vi "Init Sim Starter Kit.vi"(8 "error in (no error)":errorcluster, 10 "robot ID":string, 11 "sim starter hit host in":refnum<class "NI_Robotics_Starter Kit Host_Sim.lvclass">) -> (0 "error out":errorcluster, 3 "sim starter hit host out":refnum<class "NI_Robotics_Starter Kit Host_Sim.lvclass">)   [LabVIEW 2017, in "NI_Robotics_Starter Kit Host_Sim.lvclass"]
uses:
  <vilib>/robotics/Starter Kit/Sim Host Interface/NI_Robotics_Starter Kit Host_Sim.lvclass
  c:/Program Files (x86)/National Instruments/LabVIEW 2017/vi.lib/robotics/Starter Kit/Host Interface/NI_Robotics_Starter Kit Host.lvclass
  <vilib>/robotics/Simulator/Engine/ctl/DeviceID.ctl
  <vilib>/robotics/Starter Kit/Sim Direct IO/NI_Robotics_Starter Kit Direct IO_Sim.lvclass
  c:/Program Files (x86)/National Instruments/LabVIEW 2017/vi.lib/robotics/Starter Kit/Direct IO/NI_Robotics_Starter Kit Direct IO.lvclass
  <vilib>/robotics/Starter Kit/Host Interface/NI_Robotics_Starter Kit Host.lvclass/NI_Robotics_Starter Kit Host.ctl
  <vilib>/robotics/Starter Kit/Host Interface/NI_Robotics_Starter Kit Host.lvclass
  <vilib>/robotics/Utilities/NI_Robotics Utilities.lvlib
  <instrlib>/DC Motor Controller/HAIOL/Simulator/DC Motor Controller Simulator.lvclass
  <vilib>/robotics/Simulator/NI_Robotics_Simulator.lvlib
  <instrlib>/Parallax PING)))/HAIOL/Simulator/Parallax PING))) Simulator.lvclass
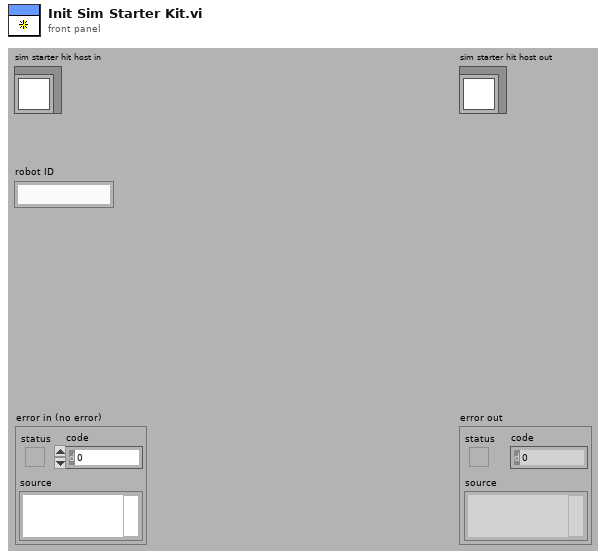
[diagram p1: front panel]
types:
  T1 = typedef "NI_Robotics_Simulator.lvlib/DeviceID.ctl" = cluster{"robot ID":string, "sensor/actuator ID":string}
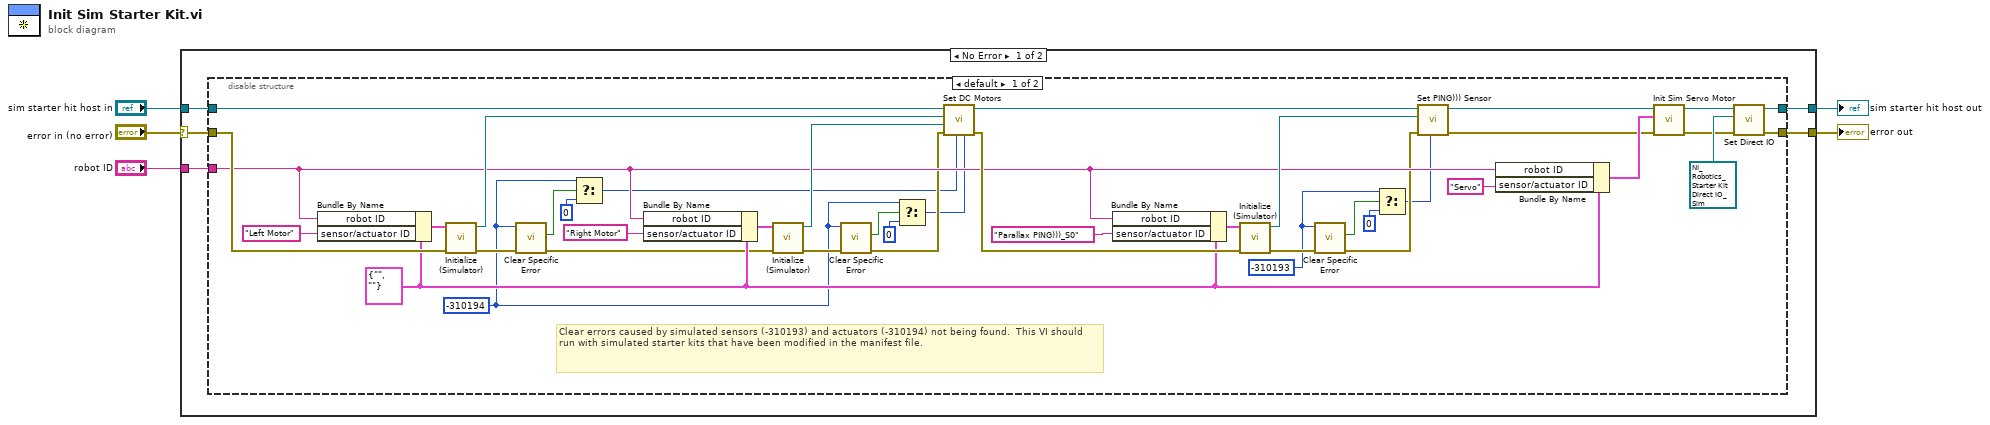
[diagram p0: block diagram]
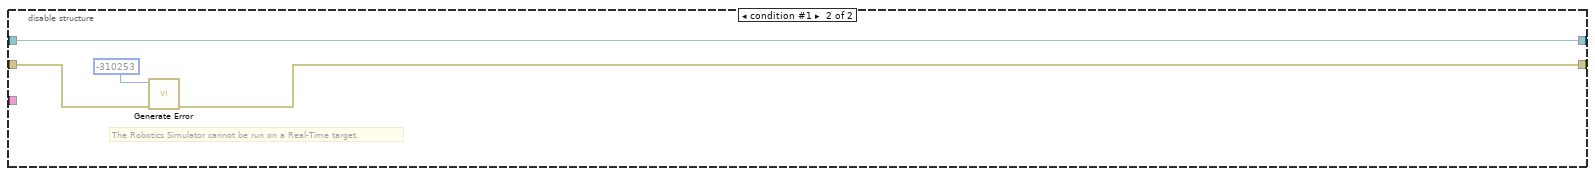
[diagram p2: hidden frame]
diagram:
  n1 = case shown="No Error" "error in (no error)" {
    selector: "error in (no error)" -> [w10 w57]
    tunnel: [w6 w57] -> w4
    tunnel: [w8 w56] -> w3
    tunnel: "sim starter hit host in" -> [w9 w56]
    tunnel: "robot ID" -> [w7 _]
    frame No Error {
      n2 = disable-structure shown="default" {
        disable-tunnel: w10 -> [w42 w54]
        disable-tunnel: w9 -> [w51 w55]
        disable-tunnel: [w32 w55] -> w8
        disable-tunnel: w7 -> [w35 _]
        disable-tunnel: [w31 w53] -> w6
        frame condition #0 (active) {
          w12 = -310193 ("code")
          w16 = -310194 ("code")
          w36 = T1 {"robot ID"="", "sensor/actuator ID"=""} ("Device ID")
          # "Clear errors caused by simulated sensors (-310193) and actuators (-310194) not being found.  This VI should run with simulated starter kits that have been modified in the manifest file."
          n3 = Bundle By Name(cluster=w36, "robot ID"=w35, "sensor/actuator ID"="Left Motor") -> (w47:T1)
          n4 = call <instrlib>:"Initialize (Simulator).vi"("error in (no error)"=w42, "Device ID"=w47) -> ("error out"=w28:errorcluster, "DC Motor Controller out"=w48:refnum<class "DC Motor Controller.lvclass">)  [unwired: 8 in]
          n5 = call <vilib>:"Clear Specific Error.vi"("error in (no error)"=w28, "code"=w16) -> ("error out"=w27:errorcluster, "cleared?"=w21:bool)  [unwired: 7 in, 1 out]
          n6 = Select(t=w16, s=w21, f=0) -> (s? t:f=w20:i32)
          n7 = Bundle By Name(cluster=w36, "robot ID"=w35, "sensor/actuator ID"="Right Motor") -> (w44:T1)
          n8 = call <instrlib>:"Initialize (Simulator).vi"("error in (no error)"=w27, "Device ID"=w44) -> ("error out"=w26:errorcluster, "DC Motor Controller out"=w45:refnum<class "DC Motor Controller.lvclass">)  [unwired: 8 in]
          n9 = call <vilib>:"Clear Specific Error.vi"("error in (no error)"=w26, "code"=w16) -> ("error out"=w25:errorcluster, "cleared?"=w18:bool)  [unwired: 7 in, 1 out]
          n10 = Select(t=w16, s=w18, f=0) -> (s? t:f=w15:i32)
          n11 = call <vilib>:"Set DC Motors.vi"("DC motor 1 error (0)"=w15, "DC motor 0 error (0)"=w20, "error in (no error)"=w25, "DC motor 1 (right)"=w45, "DC motor 0 (left)"=w48, "NI_Robotics_Starter Kit Host in"=w51) -> ("error out"=w38:errorcluster, "NI_Robotics_Starter Kit Host out"=w49:refnum<class "NI_Robotics_Starter Kit Host_Sim.lvclass">)  [unwired: 4 in]
          n12 = Bundle By Name(cluster=w36, "robot ID"=w35, "sensor/actuator ID"="Parallax PING)))_S0" ("PING))) ID")) -> (w39:T1)
          n13 = call <instrlib>:"Initialize (Simulator).vi"("error in (no error)"=w38, "Device ID"=w39) -> ("error out"=w24:errorcluster, "Parallax PING))) out"=w41:refnum<class "Parallax PING))).lvclass">)  [unwired: 8 in]
          n14 = call <vilib>:"Clear Specific Error.vi"("error in (no error)"=w24, "code"=w12) -> ("error out"=w23:errorcluster, "cleared?"=w13:bool)  [unwired: 7 in, 1 out]
          n15 = Select(t=w12, s=w13, f=0) -> (s? t:f=w11:i32)
          n16 = call <vilib>:"Set PING))) Sensor.vi"("PING))) sensor error (0)"=w11, "error in (no error)"=w23, "PING)))"=w41, "NI_Robotics_Starter Kit Host in"=w49) -> ("error out"=w29:errorcluster, "NI_Robotics_Starter Kit Host out"=w50:refnum<class "NI_Robotics_Starter Kit Host_Sim.lvclass">)  [unwired: 6 in]
          n17 = Bundle By Name(cluster=w36, "robot ID"=w35, "sensor/actuator ID"="Servo") -> (w37:T1)
          n18 = call-dynamic "Init Sim Servo Motor.vi"("error in (no error)"=w29, "device ID"=w37, "NI_Robotics_Starter Kit Host_Sim in"=w50) -> ("error out"=w22:errorcluster, "NI_Robotics_Starter Kit Host_Sim out"=w33:refnum<class "NI_Robotics_Starter Kit Host_Sim.lvclass">)  [unwired: 7 in]
          n19 = call <vilib>:"Set Direct IO.vi"("error in (no error)"=w22, "direct IO"=refnum<class "NI_Robotics_Starter Kit Direct IO_Sim.lvclass"> refnum ("NI_Robotics_Starter Kit Direct IO_Sim.lvclass"), "NI_Robotics_Starter Kit Host in"=w33) -> ("error out"=w31:errorcluster, "NI_Robotics_Starter Kit Host out"=w32:refnum<class "NI_Robotics_Starter Kit Host_Sim.lvclass">)  [unwired: 7 in]
        }
        frame condition #1 {
          # "The Robotics Simulator cannot be run on a Real-Time target."
          n20 = call <vilib>:"Generate Error.vi"("error in (no error)"=w54, "code"=-310253) -> ("error out"=w53:errorcluster)  [unwired: 9 in]
        }
      }
    }
    frame Error {
    }
  }
  "error out" <- w4
  "sim starter hit host out" <- w3
